vi "Device Under Test Tester.vi"() -> ()   [LabVIEW 2020]
uses:
  <vilib>/Utility/miscctls.llb/LVStringsAndValuesArrayTypeDef_I32.ctl
  <vilib>/Astemes/Triarc Framework/Application/Application.lvclass
  C:/Program Files (x86)/National Instruments/LabVIEW 2020/vi.lib/Astemes/Triarc Framework/Process/Process.lvclass
  <vilib>/Astemes/Triarc Framework/Process/Process.lvclass/Process.ctl
  Device Under Test/Device Under Test.lvclass
  <vilib>/Astemes/Triarc Framework/Application/Application.lvclass/Application.ctl
  <vilib>/Astemes/Triarc Framework/View/View.lvclass
  <vilib>/Astemes/Triarc Framework/View/View.lvclass/View.ctl
  <vilib>/Astemes/Triarc Framework/Process/Public/Lifecycle/Get Lifecycle State.vi
  <vilib>/Astemes/Triarc Framework/Application/Private/Retrieve Process from App.vi
  <vilib>/Astemes/Triarc Framework/Application/Private/Parse Process Name.vi
  <vilib>/Astemes/Triarc Framework/Application/Private/Get Process from Map.vi
  <vilib>/Astemes/Triarc Framework/Application/Private/Add Process to Map.vi
  <vilib>/Astemes/Triarc Framework/Application/Private/Throw Error If Process Already in App.vi
  <vilib>/Astemes/Triarc Framework/Process/Protected/Messaging/Send Message.vi
  <vilib>/Astemes/Triarc Framework/Process/Protected/SubVIs/Set Context.vi
  <vilib>/Astemes/Triarc Framework/Process/Protected/Messaging/Request Message.vi
  <vilib>/Astemes/Triarc Framework/View/Public/Get View VI Reference.vi
  <vilib>/Utility/error.llb/Clear Errors.vi
  <vilib>/Astemes/Triarc Framework/Application/Private/Remove Process from Map.vi
  <vilib>/Astemes/Triarc Framework/Process/Private/SubVIs/Wait for finish.vi
  <vilib>/Astemes/Triarc Framework/Process/Private/SubVIs/Set Lifecycle State.vi
  <vilib>/AdvancedString/Delimited String to 1D String Array.vi
  <vilib>/Astemes/Triarc Framework/Process/Private/SubVIs/Handle Debug Data.vi
  <vilib>/Astemes/Triarc Framework/Process/Public/Lifecycle/Leave Process Loop.vi
  <vilib>/Astemes/Triarc Framework/Process/Private/SubVIs/Enqueue Request Message.vi
  <vilib>/Utility/High Resolution Relative Seconds.vi
  <vilib>/Utility/error.llb/Error Cluster From Error Code.vi
  <vilib>/Astemes/Triarc Framework/Process/Private/SubVIs/Wait for Response Message.vi
  <vilib>/Astemes/Triarc Framework/Application/Protected/Get Broadcast Events Recursively.vi
  <vilib>/Astemes/Triarc Framework/Process/Process.lvclass
panel:
  out "timed out?":bool
  in  "Update DUT Status":bool
  out "Self Test Result":bool
  out "Power State":bool
  in  "Self Test":bool
  in  "Power Off":bool
  in  "Power On":bool
  in  "Refresh Modules":bool
  out "Active Modules":string[](array[string])
  in  "Stop Module":bool
  in  "Select Module":i32(ring)=-1 caption="Select Module\nTo send Request to" items=["All"=-1, "DUT 0"=0, "DUT 1"=1, "DUT 2"=2]
  in  "Run New Module":bool
  in  "Hide Module Panel":bool
  in  "Show Module Panel":bool
  out "Status":string
  # "This VI tests the API for the Module."
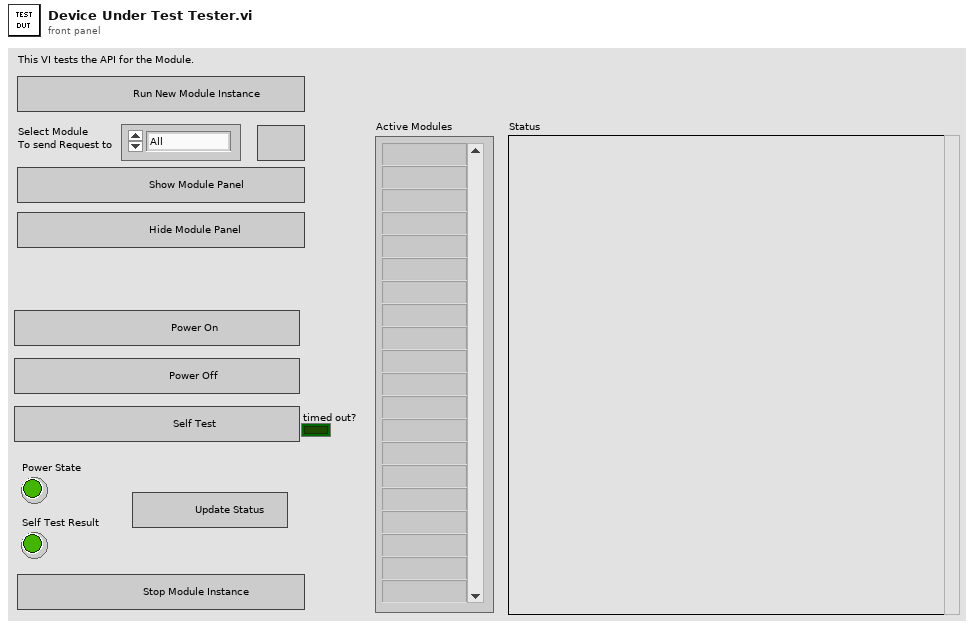
[diagram p1: front panel]
types:
  T1 = typedef "LVStringsAndValuesArrayTypeDef_I32.ctl" = cluster{"String":string, "Value":i32}[]
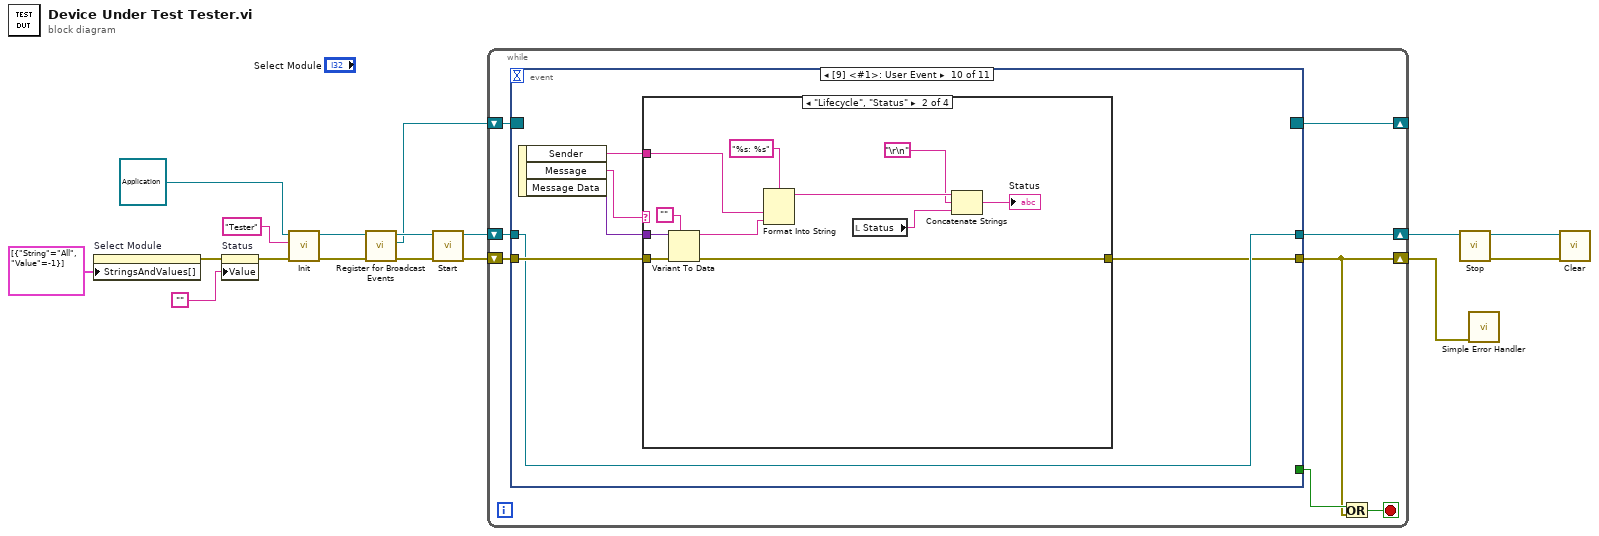
[diagram p0: block diagram]
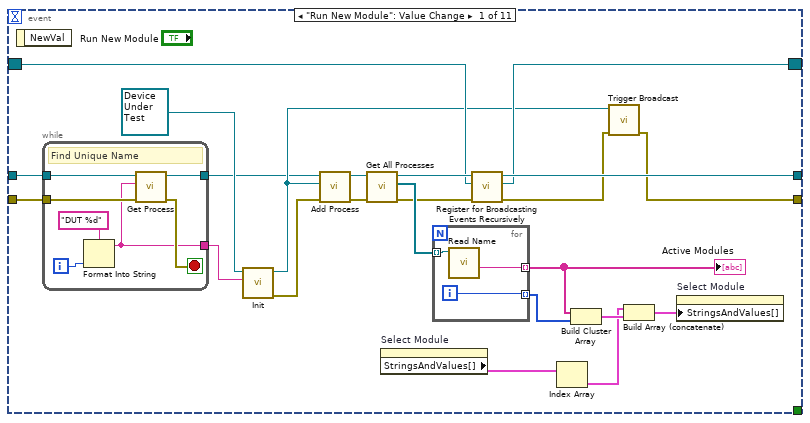
[diagram p2: hidden frame]
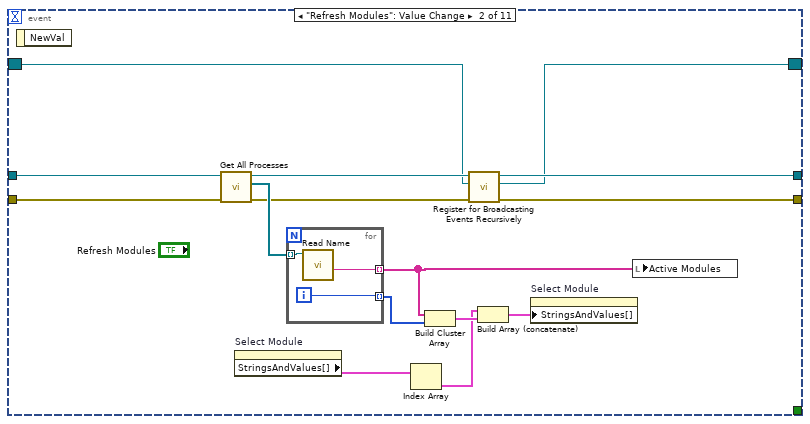
[diagram p3: hidden frame]
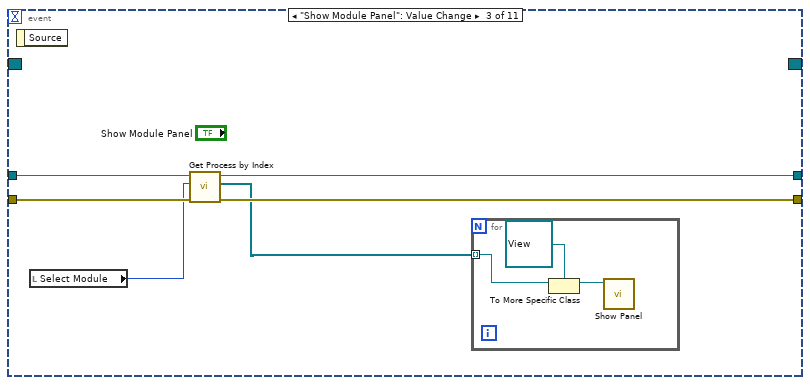
[diagram p4: hidden frame]
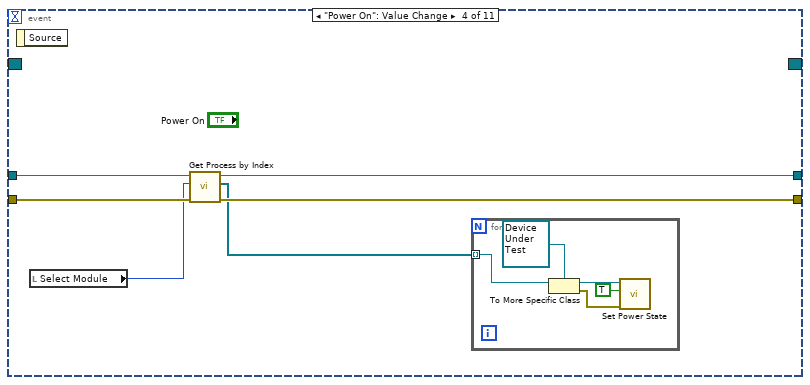
[diagram p5: hidden frame]
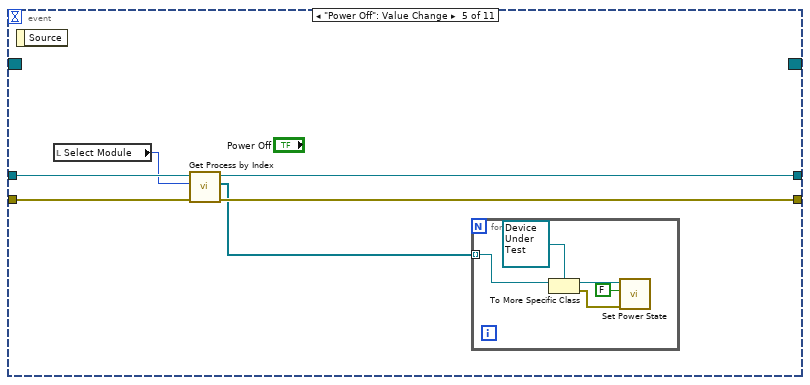
[diagram p6: hidden frame]
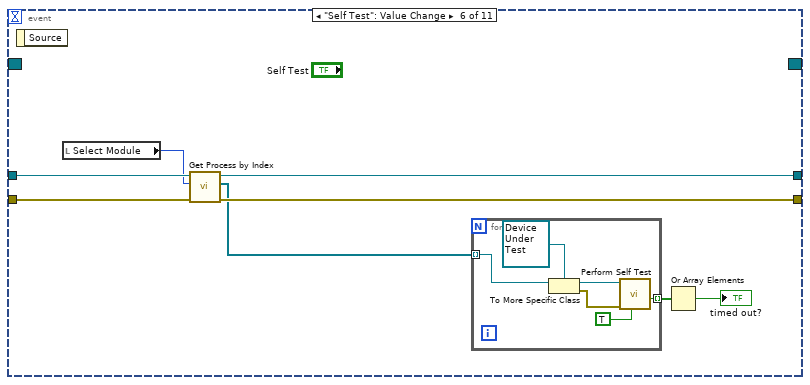
[diagram p7: hidden frame]
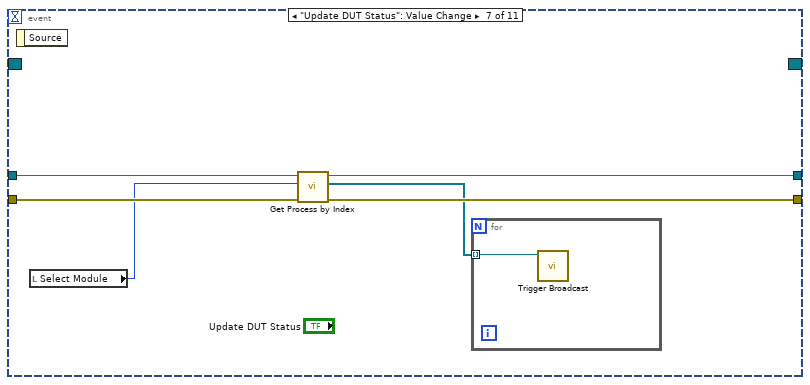
[diagram p8: hidden frame]
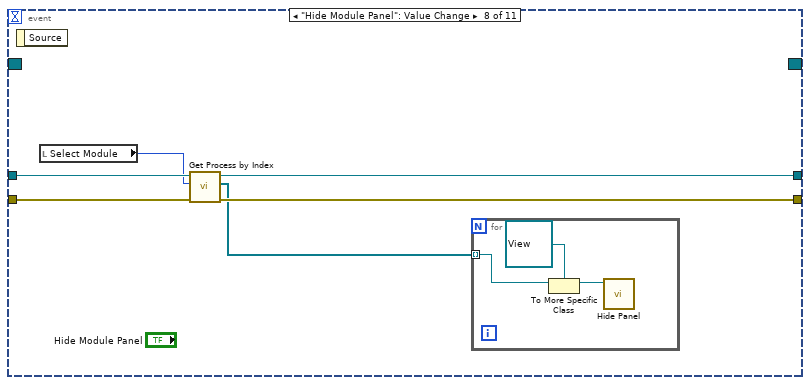
[diagram p9: hidden frame]
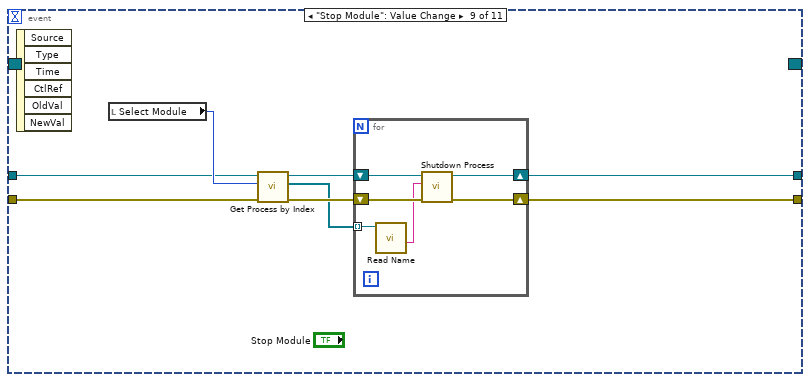
[diagram p10: hidden frame]
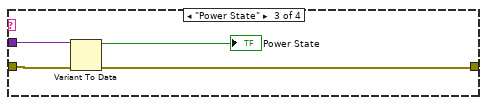
[diagram p12: hidden frame]
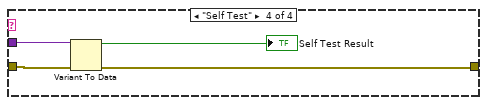
[diagram p13: hidden frame]
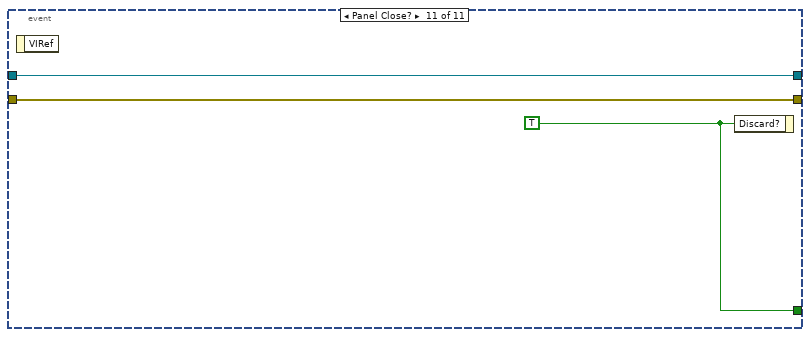
[diagram p14: hidden frame]
diagram:
  n1 = property on="Select Module" class="Ring (strict)"("StringsAndValues[]"=T1 [{"String"="All", "Value"=-1}] ("Strings And Values []")) -> (error out=w3:errorcluster)  [unwired: 2 in, 1 out]
  n2 = property on="Status" class="Str"(error in=w3, "Value"="") -> (error out=w2:errorcluster)  [unwired: 1 in, 1 out]
  n3 = call-dynamic "Init.vi"("error in (no error)"=w2, "Name"="Tester", "Process In"=refnum<class "Application.lvclass"> refnum ("TF.lvlib:Application.lvclass")) -> ("error out"=w4:errorcluster, "Process Out"=w8:refnum<class "Application.lvclass">)  [unwired: 7 in]
  n4 = call <vilib>:"Register for Broadcast Events.vi"("error in (no error)"=w4, "Process In"=w8) -> ("error out"=w6:errorcluster, "Event Registration Refnum Out"=w5:refnum<event-registration>, "Process Out"=w7:refnum<class "Application.lvclass">)  [unwired: 7 in]
  n5 = call <vilib>:"Start.vi"("error in (no error)"=w6, "Process In"=w7) -> ("error out"=w13:errorcluster, "Process Out"=w11:refnum<class "Application.lvclass">)  [unwired: 7 in, 1 out]
  n6 = while {
    shift-right: [w22] -> w17
    shift-left: w13 -> [w25]
    shift-right: [w20] -> w16
    shift-left: w11 -> [w21]
    shift-right: [w18] -> _
    shift-left: w5 -> [w19]
    stop <- w23 stop-if-true
    n7 = event shown="[9] <#1>: User Event" {
      selector: w19 -> [w33 w59 _ _ _ _ _ _ _ _ _]
      dyn-events: [w34 w60 _ _ _ _ _ _ _ _ _] -> w18
      timeout: _ -> [_ _ _ _ _ _ _ _ _ _ _]
      tunnel: w25 -> [w29 w68 w82 w91 w102 w115 w127 w134 w143 w156 w179]
      tunnel: [w30 w62 w81 w90 w101 w114 w126 w133 w139 w152 w179] -> w22
      tunnel: [_ _ _ _ _ _ _ _ _ _ w180] -> w24
      tunnel: w21 -> [w28 w67 w80 w89 w100 w113 w125 w132 w144 w154 w178]
      tunnel: [w36 w63 w79 w88 w99 w112 w124 w131 w140 w154 w178] -> w20
      event "Run New Module": Value Change {
        n8 = event-data() -> ()  [unwired: 1 in, 1 out]
        n9 = while {
          tunnel: w29 -> [w54]
          tunnel: w28 -> [w53]
          tunnel: [w52] -> w27
          tunnel: [w49] -> w26
          i -> [w51]
          stop <- w50 stop-if-true
          # "Find Unique Name"
          n10 = Format Into String(format string="DUT %d", w51) -> (resulting string=w49:string)  [unwired: 2 in, 1 out]
          n11 = call <vilib>:"Get Process.vi"("error in (no error)"=w54, "Process Name"=w49, "Application In"=w53) -> ("error out"=w50:errorcluster, "Application Out"=w52:refnum<class "Application.lvclass">)  [unwired: 6 in, 1 out]
        }
        n12 = call-dynamic "Init.vi"("Name"=w26, "View In"=refnum<class "Device Under Test.lvclass"> refnum ("Device Under Test.lvclass")) -> ("error out"=w41:errorcluster, "View Out"=w32:refnum<class "Device Under Test.lvclass">)  [unwired: 8 in]
        n13 = call <vilib>:"Add Process.vi"("error in (no error)"=w41, "Process"=w32, "Application In"=w27) -> ("error out"=w39:errorcluster, "Application Out"=w40:refnum<class "Application.lvclass">)  [unwired: 7 in]
        n14 = call <vilib>:"Get All Processes.vi"("error in (no error)"=w39, "Application In"=w40) -> ("error out"=w35:errorcluster, "App Processes"=w38:refnum<class "Process.lvclass">[], "Application Out"=w37:refnum<class "Application.lvclass">)  [unwired: 7 in]
        n15 = property on="Select Module" class="Ring (strict)"() -> ("StringsAndValues[]"=w44:T1)  [unwired: 2 in, 2 out]
        n16 = for {
          tunnel: [w56] -> w47 mode=indexing
          tunnel: [w58] -> w46 mode=indexing
          tunnel: w38 -> [w57] mode=indexing
          i -> [w58]
          n17 = call <vilib>:"Read Name.vi"("Process In"=w57) -> ("Name"=w56:string)  [unwired: 7 in, 3 out]
        }
        "Active Modules" <- w47
        n18 = call <vilib>:"Register for Broadcasting Events Recursively.vi"("error in (no error)"=w35, "Event Registration Refnum In"=w33, "Application In"=w37) -> ("error out"=w31:errorcluster, "Event Registration Refnum Out"=w34:refnum<event-registration>, "Application Out"=w36:refnum<class "Application.lvclass">)  [unwired: 6 in]
        n19 = Index Array(array=w44) -> (element=w42:cluster{"String":string, "Value":i32})  [unwired: 1 in]
        n20 = Build Cluster Array(w47, w46) -> (w45:cluster{"Name":string, i32}[])
        n21 = call <vilib>:"Trigger Broadcast.vi"("error in (no error)"=w31, "Process in"=w32) -> ("error out"=w30:errorcluster)  [unwired: 8 in, 1 out]
        n22 = Build Array (concatenate)(w42, w45) -> (w43:cluster{"Name":string, "Value":i32}[])
        n23 = property on="Select Module" class="Ring (strict)"("StringsAndValues[]"=w43) -> ()  [unwired: 2 in, 2 out]
      }
      event "Refresh Modules": Value Change {
        n24 = event-data() -> ()  [unwired: 1 in, 1 out]
        n25 = call <vilib>:"Get All Processes.vi"("error in (no error)"=w68, "Application In"=w67) -> ("error out"=w61:errorcluster, "App Processes"=w66:refnum<class "Process.lvclass">[], "Application Out"=w64:refnum<class "Application.lvclass">)  [unwired: 7 in]
        n26 = property on="Select Module" class="Ring (strict)"() -> ("StringsAndValues[]"=w71:T1)  [unwired: 2 in, 2 out]
        n27 = for {
          tunnel: [w74] -> w65 mode=indexing
          tunnel: [w76] -> w73 mode=indexing
          tunnel: w66 -> [w75] mode=indexing
          i -> [w76]
          n28 = call <vilib>:"Read Name.vi"("Process In"=w75) -> ("Name"=w74:string)  [unwired: 7 in, 3 out]
        }
        n29 = Index Array(array=w71) -> (element=w69:cluster{"String":string, "Value":i32})  [unwired: 1 in]
        n30 = Build Cluster Array(w65, w73) -> (w72:cluster{"Name":string, i32}[])
        n31 = call <vilib>:"Register for Broadcasting Events Recursively.vi"("error in (no error)"=w61, "Event Registration Refnum In"=w59, "Application In"=w64) -> ("error out"=w62:errorcluster, "Event Registration Refnum Out"=w60:refnum<event-registration>, "Application Out"=w63:refnum<class "Application.lvclass">)  [unwired: 6 in]
        n32 = Build Array (concatenate)(w69, w72) -> (w70:cluster{"Name":string, "Value":i32}[])
        n33 = property on="Select Module" class="Ring (strict)"("StringsAndValues[]"=w70) -> ()  [unwired: 2 in, 2 out]
        n34 = local write "Active Modules"(w65) -> ()
      }
      event "Show Module Panel": Value Change {
        n35 = event-data() -> ()  [unwired: 1 in, 1 out]
        n36 = local read "Select Module"() -> (w78:i32)
        n37 = call "Get Process by Index.vi"("error in (no error)"=w82, "Select Module"=w78, "Application in"=w80) -> ("error out"=w81:errorcluster, "Processes"=w77:refnum<class "Process.lvclass">[], "Application out"=w79:refnum<class "Application.lvclass">)  [unwired: 6 in]
        n38 = for {
          tunnel: w77 -> [w85] mode=indexing
          n39 = To More Specific Class(target class=refnum<class "View.lvclass"> refnum ("View In"), reference=w85) -> (specific class reference=w84:refnum<class "View.lvclass">)  [unwired: 1 in, 1 out]
          n40 = call <vilib>:"Show Panel.vi"("View In"=w84) -> ()  [unwired: 9 in, 2 out]
        }
      }
      event "Power On": Value Change {
        n41 = event-data() -> ()  [unwired: 1 in, 1 out]
        n42 = local read "Select Module"() -> (w86:i32)
        n43 = call "Get Process by Index.vi"("error in (no error)"=w91, "Select Module"=w86, "Application in"=w89) -> ("error out"=w90:errorcluster, "Processes"=w87:refnum<class "Process.lvclass">[], "Application out"=w88:refnum<class "Application.lvclass">)  [unwired: 6 in]
        n44 = for {
          tunnel: w87 -> [w96] mode=indexing
          n45 = To More Specific Class(target class=refnum<class "Device Under Test.lvclass"> refnum ("Device Under Test Out"), reference=w96) -> (specific class reference=w95:refnum<class "Device Under Test.lvclass">, error out=w93:errorcluster)  [unwired: 1 in]
          n46 = call "Set Power State.vi"("error in (no error)"=w93, "Power State"=TRUE, "Device Under Test In"=w95) -> ()  [unwired: 7 in, 2 out]
        }
      }
      event "Power Off": Value Change {
        n47 = event-data() -> ()  [unwired: 1 in, 1 out]
        n48 = local read "Select Module"() -> (w97:i32)
        n49 = call "Get Process by Index.vi"("error in (no error)"=w102, "Select Module"=w97, "Application in"=w100) -> ("error out"=w101:errorcluster, "Processes"=w98:refnum<class "Process.lvclass">[], "Application out"=w99:refnum<class "Application.lvclass">)  [unwired: 6 in]
        n50 = for {
          tunnel: w98 -> [w107] mode=indexing
          n51 = To More Specific Class(target class=refnum<class "Device Under Test.lvclass"> refnum ("Device Under Test Out"), reference=w107) -> (specific class reference=w106:refnum<class "Device Under Test.lvclass">, error out=w104:errorcluster)  [unwired: 1 in]
          n52 = call "Set Power State.vi"("error in (no error)"=w104, "Power State"=FALSE, "Device Under Test In"=w106) -> ()  [unwired: 7 in, 2 out]
        }
      }
      event "Self Test": Value Change {
        n53 = event-data() -> ()  [unwired: 1 in, 1 out]
        n54 = local read "Select Module"() -> (w108:i32)
        n55 = call "Get Process by Index.vi"("error in (no error)"=w115, "Select Module"=w108, "Application in"=w113) -> ("error out"=w114:errorcluster, "Processes"=w111:refnum<class "Process.lvclass">[], "Application out"=w112:refnum<class "Application.lvclass">)  [unwired: 6 in]
        n56 = for {
          tunnel: w111 -> [w121] mode=indexing
          tunnel: [w116] -> w110 mode=indexing
          n57 = To More Specific Class(target class=refnum<class "Device Under Test.lvclass"> refnum ("Device Under Test Out"), reference=w121) -> (specific class reference=w120:refnum<class "Device Under Test.lvclass">, error out=w118:errorcluster)  [unwired: 1 in]
          n58 = call "Perform Self Test.vi"("Wait for Reply?"=TRUE, "error in (no error)"=w118, "Device Under Test In"=w120) -> ("Timed out?"=w116:bool)  [unwired: 5 in, 3 out]
        }
        n59 = Or Array Elements(Boolean array=w110) -> (logical OR=→"timed out?":bool)
      }
      event "Update DUT Status": Value Change {
        n60 = event-data() -> ()  [unwired: 1 in, 1 out]
        n61 = local read "Select Module"() -> (w122:i32)
        n62 = call "Get Process by Index.vi"("error in (no error)"=w127, "Select Module"=w122, "Application in"=w125) -> ("error out"=w126:errorcluster, "Processes"=w123:refnum<class "Process.lvclass">[], "Application out"=w124:refnum<class "Application.lvclass">)  [unwired: 6 in]
        n63 = for {
          tunnel: w123 -> [w128] mode=indexing
          n64 = call <vilib>:"Trigger Broadcast.vi"("Process in"=w128) -> ()  [unwired: 9 in, 2 out]
        }
      }
      event "Hide Module Panel": Value Change {
        n65 = event-data() -> ()  [unwired: 1 in, 1 out]
        n66 = local read "Select Module"() -> (w129:i32)
        n67 = call "Get Process by Index.vi"("error in (no error)"=w134, "Select Module"=w129, "Application in"=w132) -> ("error out"=w133:errorcluster, "Processes"=w130:refnum<class "Process.lvclass">[], "Application out"=w131:refnum<class "Application.lvclass">)  [unwired: 6 in]
        n68 = for {
          tunnel: w130 -> [w137] mode=indexing
          n69 = To More Specific Class(target class=refnum<class "View.lvclass"> refnum ("View In"), reference=w137) -> (specific class reference=w136:refnum<class "View.lvclass">)  [unwired: 1 in, 1 out]
          n70 = call <vilib>:"Hide Panel.vi"("View In"=w136) -> ()  [unwired: 9 in, 2 out]
        }
      }
      event "Stop Module": Value Change {
        n71 = event-data() -> ()  [unwired: 1 in, 6 out]
        n72 = local read "Select Module"() -> (w145:i32)
        n73 = call "Get Process by Index.vi"("error in (no error)"=w143, "Select Module"=w145, "Application in"=w144) -> ("error out"=w142:errorcluster, "Processes"=w138:refnum<class "Process.lvclass">[], "Application out"=w141:refnum<class "Application.lvclass">)  [unwired: 6 in]
        n74 = for {
          shift-right: [w148] -> w139
          shift-left: w142 -> [w151]
          shift-right: [w149] -> w140
          shift-left: w141 -> [w150]
          tunnel: w138 -> [w147] mode=indexing
          n75 = call <vilib>:"Read Name.vi"("Process In"=w147) -> ("Name"=w146:string)  [unwired: 7 in, 3 out]
          n76 = call <vilib>:"Shutdown Process.vi"("error in (no error)"=w151, "Process Name"=w146, "Application In"=w150) -> ("error out"=w148:errorcluster, "Application Out"=w149:refnum<class "Application.lvclass">)  [unwired: 7 in]
        }
      }
      event User Event {
        n77 = event-data() -> ("Sender"=w153:string, "Message"=w157:string, "Message Data"=w155:variant)  [unwired: 1 in]
        n78 = case shown="\"Lifecycle\", \"Status\"" w157 {
          tunnel: w156 -> [w158 w169 w172 w176]
          tunnel: w155 -> [_ w168 w173 w177]
          tunnel: w153 -> [_ w166 _ _]
          tunnel: [w158 w163 w170 w175] -> w152
          frame Default {
          }
          frame "Lifecycle", "Status" {
            n79 = Variant To Data(error in=w169, type="", Variant=w168) -> (data=w165:string, error out=w163:errorcluster)
            n80 = Format Into String(format string="%s: %s", w166, w165) -> (resulting string=w160:string)  [unwired: 2 in, 1 out]
            n81 = local read "Status"() -> (w162:string)
            n82 = Concatenate Strings(w160, "\r\n", w162) -> (→"Status":string)
          }
          frame "Power State" {
            n83 = Variant To Data(error in=w172, Variant=w173) -> (data=→"Power State":bool, error out=w170:errorcluster)  [unwired: 1 in]
          }
          frame "Self Test" {
            n84 = Variant To Data(error in=w176, Variant=w177) -> (data=→"Self Test Result":bool, error out=w175:errorcluster)  [unwired: 1 in]
          }
        }
      }
      event Panel Close? {
        w180 = TRUE ("Discard?")
        n85 = event-data() -> ()  [unwired: 1 in, 1 out]
        n86 = event-data("Discard?"=w180) -> ()  [unwired: 1 in, 1 out]
      }
    }
    n87 = Or(x=w24, y=w22) -> (x .or. y?=w23:bool)
  }
  n88 = call <vilib>:"Stop.vi"("Process In"=w16) -> ("error out"=w10:errorcluster, "Process Out"=w9:refnum<class "Application.lvclass">)  [unwired: 8 in, 1 out]
  n89 = call <vilib>:"Simple Error Handler.vi"("error in (no error)"=w17) -> ()  [unwired: 4 in, 5 out]
  n90 = call-dynamic "Clear.vi"("error in (no error)"=w10, "Application In"=w9) -> ()  [unwired: 9 in, 1 out]
